vi "Sort 2D Array - Pop Stack.vi"(10 "array in":i32[](array[numeric]), 11 "top in":i32) -> (1 "element":i32, 2 "array out":i32[](array[numeric]), 3 "top out":i32)   [LabVIEW 2017]
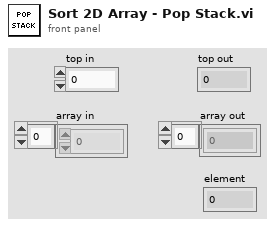
[diagram p1: front panel]
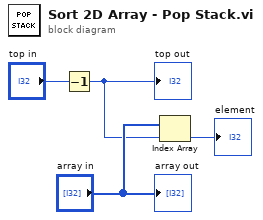
[diagram p0: block diagram]
diagram:
  n1 = Decrement(x="top in") -> (x-1=w1:i32)
  "top out" <- w1
  n2 = Index Array(array="array in", index=w1) -> (element=→"element":i32)
  "array out" <- "array in"
